vi "Vi Tree.vi"   [LabVIEW 2020, in "LV Process library.lvlib"]
doc: "List of all VIs of LV Process library.\n\n---\nLV Process works only with lv_proc.dll library, which is part of vipm package or should be delivered together with packed library. Placement of this dll is selected in terminal of Create Process.vi."
uses:
  LV Process library.lvlib
  Pipe Handle.ctl
types:
  T1 = typedef "LV Process library.lvlib/Pipe Handle.ctl" = cluster{"lv_proc.dll file path":path, "process instance handle":u32[], "debug mode":bool, "debug data":cluster{"time":timestamp, "stdin":bool, "data":string}[]}
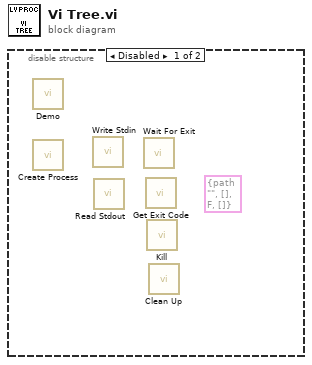
[diagram p0: block diagram]
diagram:
  n1 = disable-structure shown="Disabled" {
    frame Disabled {
      (unwired) T1 {"lv_proc.dll file path"=path "", "process instance handle"=[], "debug mode"=FALSE, "debug data"=[]} ("pipe handle")
      n2 = call "Demo.vi"() -> ()  [unwired: 12 in]
      n3 = call "Create Process.vi"() -> ()  [unwired: 10 in, 2 out]
      n4 = call "Write Stdin.vi"() -> ()  [unwired: 9 in, 3 out]
      n5 = call "Read Stdout.vi"() -> ()  [unwired: 6 in, 6 out]
      n6 = call "Wait For Exit.vi"() -> ()  [unwired: 9 in, 3 out]
      n7 = call "Get Exit Code.vi"() -> ()  [unwired: 7 in, 5 out]
      n8 = call "Kill.vi"() -> ()  [unwired: 10 in, 2 out]
      n9 = call "Clean Up.vi"() -> ()  [unwired: 11 in, 1 out]
    }
    frame Enabled {
    }
  }
